vi "UDT_admittanceLibrary_TargetMet.vi"() -> (3 "Unit Test Framework Results":T1)   [LabVIEW 2017]
doc: "Use this template to create a user-defined test VI. Define your test requirements and wire the results to the <b>Result (Test)</b> control. Do not modify the <b>Unit Test Framework Results</b> indicator."
uses:
  <vilib>/utf/common/utf_test_result_troll.ctl
  <vilib>/utf/common/utf_test_result.ctl
  <vilib>/utf/common/utf_test_result_failure.ctl
  <vilib>/utf/common/utf_test_comparison_operators.ctl
  <vilib>/utf/common/utf_vi_tag.ctl
  <vilib>/Control Software Solutions Ltd/UTF Helper/SubVIs/UTF I32 Equals.vi
  <vilib>/Control Software Solutions Ltd/UTF Helper/Unit Test Helper.lvlib
  RT/Admittance Controller/admittanceControllerLibrary.lvlib
  <vilib>/utf/NI_UnitTestFramework.lvlib
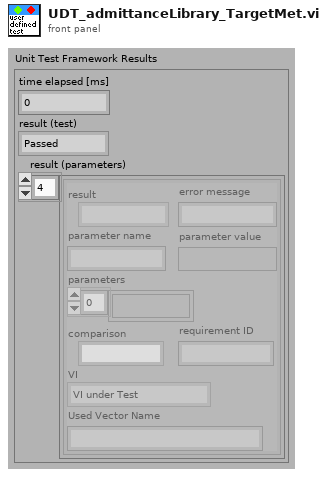
[diagram p1: front panel]
types:
  T1 = typedef "NI_UnitTestFramework.lvlib/utf_test_result_troll.ctl" = cluster{"time elapsed [ms]":u32, "result (test)":T2, "result (parameters)":T3[]}
  T2 = typedef "NI_UnitTestFramework.lvlib/utf_test_result.ctl" = enum16{"Passed", "Failed", "Error", "Skipped", "Not Processed"}
  T3 = typedef "NI_UnitTestFramework.lvlib/utf_test_result_failure.ctl" = cluster{"result":T2, "error message":string, "parameter name":string, "parameter value":variant, "parameters":variant[], "comparison":T4, "requirement ID":string, "VI":T5, "Used Vector Name":string}
  T4 = typedef "NI_UnitTestFramework.lvlib/utf_test_comparison_operators.ctl" = enum16{"=", "!=", ">", ">=", "<", "<=", "range", "symmetric tolerance", "asymmetric tolerance", "string contains", "string not contain", "array size", "string length", "array range", "by element", "array range (limit array)", "user-defined", "array contains", "array not contain", "vector length", "= (elm)", "!= (elm)", "= (case insensitive)", "!= (case insensitive)"}
  T5 = typedef "NI_UnitTestFramework.lvlib/utf_vi_tag.ctl" = enum16{"Setup VI", "VI under Test", "Teardown VI"}
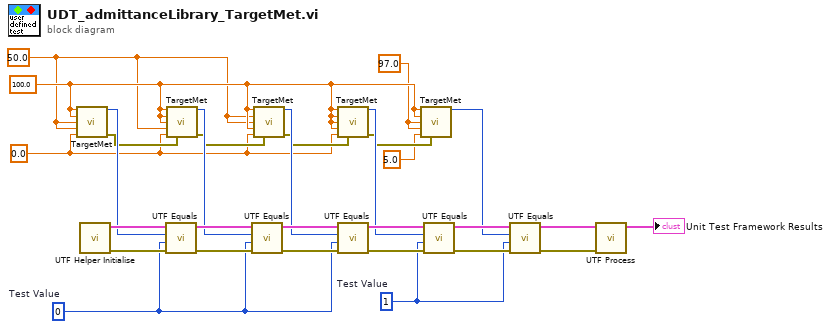
[diagram p0: block diagram]
diagram:
  w1 = 1  # Test Value
  w2 = 0  # Test Value
  w3 = 97.0
  w5 = 0.0
  w6 = 50.0
  w7 = 100.0
  n1 = call "TargetMet.vi"("Target x (mm)"=w7, "Target y (mm)"=w7, "Current x (mm)"=w6, "Current y (mm)"=w6, "Dead Zone (mm)"=w5) -> ("out"=w12:i32, "error out"=w11:errorcluster)  [unwired: 9 in]
  n2 = call <vilib>:"UTF Helper Initialise.vi"() -> ("error out"=w23:errorcluster, "results array"=w22:T3[])  [unwired: 10 in]
  n3 = call-poly <vilib>:"UTF Equals.vi"("error in (no error)"=w23, "Test Value"=w2, "Input"=w12, "Input Results"=w22) -> ("error out"=w24:errorcluster, "Output Results"=w21:T3[])  [unwired: 6 in]
  n4 = call "TargetMet.vi"("Target x (mm)"=w7, "Target y (mm)"=w7, "Current x (mm)"=w7, "Current y (mm)"=w6, "Dead Zone (mm)"=w5, "error in (no error)"=w11) -> ("out"=w13:i32, "error out"=w10:errorcluster)  [unwired: 8 in]
  n5 = call-poly <vilib>:"UTF Equals.vi"("error in (no error)"=w24, "Test Value"=w2, "Input"=w13, "Input Results"=w21) -> ("error out"=w25:errorcluster, "Output Results"=w20:T3[])  [unwired: 6 in]
  n6 = call "TargetMet.vi"("Target x (mm)"=w7, "Target y (mm)"=w6, "Current x (mm)"=w6, "Current y (mm)"=w7, "Dead Zone (mm)"=w5, "error in (no error)"=w10) -> ("out"=w14:i32, "error out"=w9:errorcluster)  [unwired: 8 in]
  n7 = call "TargetMet.vi"("Target x (mm)"=w7, "Target y (mm)"=w7, "Current x (mm)"=w7, "Current y (mm)"=w7, "Dead Zone (mm)"=w5, "error in (no error)"=w9) -> ("out"=w15:i32, "error out"=w8:errorcluster)  [unwired: 8 in]
  n8 = call-poly <vilib>:"UTF Equals.vi"("error in (no error)"=w25, "Test Value"=w2, "Input"=w14, "Input Results"=w20) -> ("error out"=w26:errorcluster, "Output Results"=w19:T3[])  [unwired: 6 in]
  n9 = call "TargetMet.vi"("Target x (mm)"=w7, "Target y (mm)"=w7, "Current x (mm)"=w3, "Current y (mm)"=w3, "Dead Zone (mm)"=5.0, "error in (no error)"=w8) -> ("out"=w16:i32)  [unwired: 8 in, 1 out]
  n10 = call-poly <vilib>:"UTF Equals.vi"("error in (no error)"=w26, "Test Value"=w1, "Input"=w15, "Input Results"=w19) -> ("error out"=w27:errorcluster, "Output Results"=w18:T3[])  [unwired: 6 in]
  n11 = call-poly <vilib>:"UTF Equals.vi"("error in (no error)"=w27, "Test Value"=w1, "Input"=w16, "Input Results"=w18) -> ("error out"=w28:errorcluster, "Output Results"=w17:T3[])  [unwired: 6 in]
  n12 = call <vilib>:"UTF Process.vi"("error in (no error)"=w28, "results array"=w17) -> ("Unit Test Framework Results"=→"Unit Test Framework Results":T1)  [unwired: 9 in]
